vi "SetContextMenu.vi"(8 "error in (no error)":errorcluster, 11 "Gviewer in":refnum<class "Gviewer.lvclass">) -> (0 "error out":errorcluster, 3 "Gviewer out":refnum<class "Gviewer.lvclass">)   [LabVIEW 2020, in "Sgraph_lib_V1.lvlib" / "Gviewer.lvclass"]
doc: "Andre Koelewijn, 5 jan 2021\n\nSet or refresh the Contect (right mouse button) context menu structure"
uses:
  Gviewer.lvclass
  Gviewer.lvclass/Gviewer.ctl
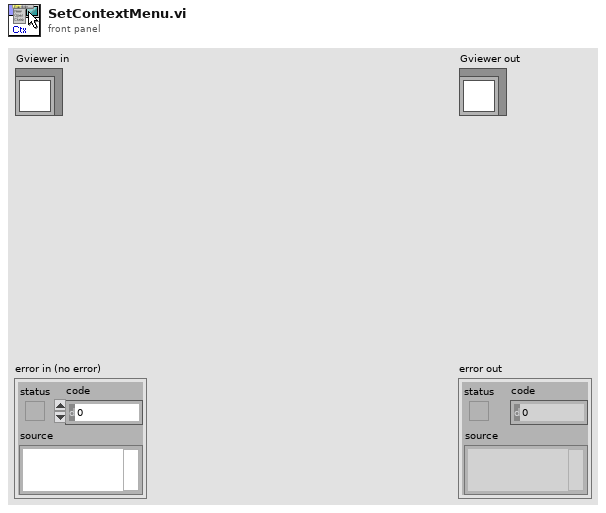
[diagram p1: front panel]
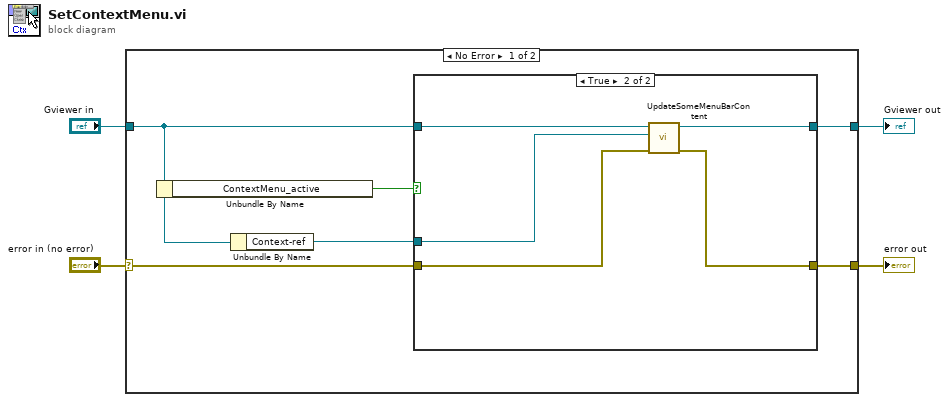
[diagram p0: block diagram]
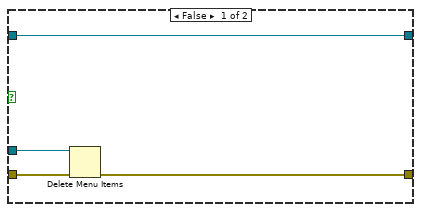
[diagram p2: hidden frame]
diagram:
  n1 = case shown="No Error" "error in (no error)" {
    selector: "error in (no error)" -> [w5 w21]
    tunnel: [w9 w21] -> w3
    tunnel: [w10 w20] -> w1
    tunnel: "Gviewer in" -> [w7 w20]
    frame No Error {
      n2 = Unbundle By Name(w7) -> ("ContextMenu_active"=w8:bool)
      n3 = Unbundle By Name(w7) -> ("Context-ref"=w6:refnum<k9>)
      n4 = case shown="True" w8 {
        tunnel: w7 -> [w14 w16]
        tunnel: [w14 w17] -> w10
        tunnel: [w11 w15] -> w9
        tunnel: w5 -> [w12 w19]
        tunnel: w6 -> [w13 w18]
        frame False {
          n5 = Delete Menu Items(6:w12, 9:w13) -> (0:w11:errorcluster)  [unwired: 2 in, 1 out]
        }
        frame True {
          n6 = call "UpdateSomeMenuBarContent.vi"("error in (no error)"=w19, "menu ref"=w18, "Gviewer in"=w16) -> ("error out"=w15:errorcluster, "Gviewer out"=w17:refnum<class "Gviewer.lvclass">)  [unwired: 7 in]
        }
      }
    }
    frame Error {
    }
  }
  "error out" <- w3
  "Gviewer out" <- w1
